vi "test.vi"() -> ()   [LabVIEW 2021]
uses:
  CParent/CParent.lvclass
  IParent/IParent.lvclass
  IBar/IBar.lvclass
panel:
  out "Numeric":dbl
  out "result":string="IParent's static method is called!"
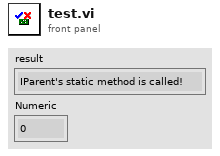
[diagram p1: front panel]
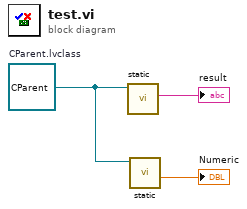
[diagram p0: block diagram]
diagram:
  w2 = refnum<class "CParent.lvclass"> refnum  # CParent.lvclass
  n1 = call "static.vi"("IParent in"=w2) -> ("result"=→"result":string)  [unwired: 8 in, 2 out]
  n2 = call "static.vi"("IBar in"=w2) -> ("Numeric"=→"Numeric":dbl)  [unwired: 8 in, 2 out]
